vi "RTS Open Delete Config File.vi"(8 "error in (no error)":errorcluster, 10 "Station Settings.Chamber Test Pattern":T2, 11 "Station Number":u16=1 min=1 max=8 step=1) -> (0 "Error Out":errorcluster, 3 "Refnum out":T1)   [LabVIEW 2016]
uses:
  Type Definitions/RTS Test Pattern.ctl
  <vilib>/Utility/config.llb/Config Data RefNum.ctl
  <vilib>/Utility/config.llb/NI_LVConfig.lvlib
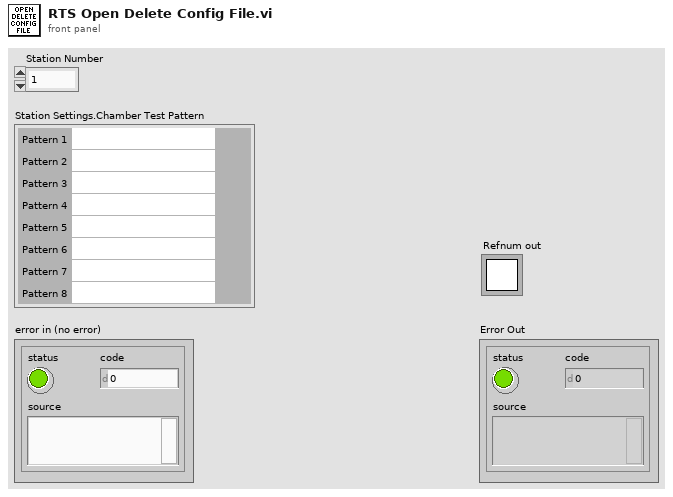
[diagram p1: front panel]
types:
  T1 = typedef "NI_LVConfig.lvlib/Config Data RefNum.ctl" = refnum<k1>
  T2 = typedef "RTS Test Pattern.ctl" = cluster{" Pattern 1":path, "Pattern 2":path, "Pattern 3":path, "Pattern 4":path, "Pattern 5":path, "Pattern 6":path, "Pattern 7":path, "Pattern 8":path}
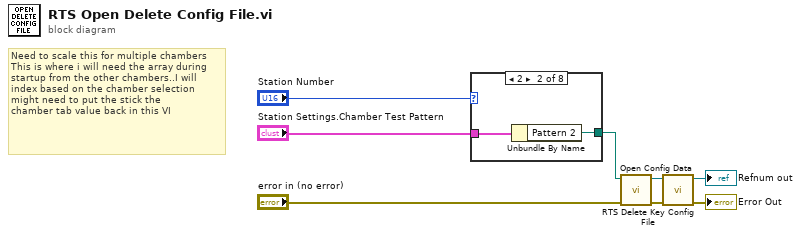
[diagram p0: block diagram]
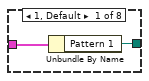
[diagram p2: hidden frame]
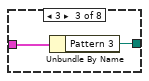
[diagram p3: hidden frame]
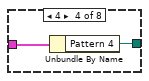
[diagram p4: hidden frame]
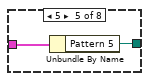
[diagram p5: hidden frame]
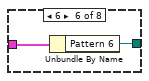
[diagram p6: hidden frame]
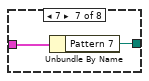
[diagram p7: hidden frame]
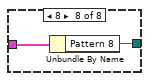
[diagram p8: hidden frame]
diagram:
  # "Need to scale this for multiple chambers\nThis is where i will need the array during\nstartup from the other chambers..I will\nindex based on the chamber selection\nmight need to put the stick the \nchamber tab value back in this VI"
  n1 = case shown="2" "Station Number" {
    tunnel: "Station Settings.Chamber Test Pattern" -> [w10 w12 w14 w16 w18 w20 w22 w24]
    tunnel: [w9 w11 w13 w15 w17 w19 w21 w23] -> w4
    frame 1, Default {
      n2 = Unbundle By Name(w10) -> ("Pattern 1"=w9:path)
    }
    frame 2 {
      n3 = Unbundle By Name(w12) -> ("Pattern 2"=w11:path)
    }
    frame 3 {
      n4 = Unbundle By Name(w14) -> ("Pattern 3"=w13:path)
    }
    frame 4 {
      n5 = Unbundle By Name(w16) -> ("Pattern 4"=w15:path)
    }
    frame 5 {
      n6 = Unbundle By Name(w18) -> ("Pattern 5"=w17:path)
    }
    frame 6 {
      n7 = Unbundle By Name(w20) -> ("Pattern 6"=w19:path)
    }
    frame 7 {
      n8 = Unbundle By Name(w22) -> ("Pattern 7"=w21:path)
    }
    frame 8 {
      n9 = Unbundle By Name(w24) -> ("Pattern 8"=w23:path)
    }
  }
  n10 = call <vilib>:"Open Config Data.vi"("error in (no error)"="error in (no error)", "configuration file path"=w4) -> ("error out"=w7:errorcluster, "refnum"=w8:T1)  [unwired: 1 in, 7 out]
  n11 = call "RTS Delete Key Config File.vi"("error in (no error)"=w7, "Refnum in"=w8) -> ("error out"=→"Error Out":errorcluster, "Refnum out"=→"Refnum out":T1)  [unwired: 8 in]
